vi "Interpolate 2D Scattered_Gradient.vi"(0 "X(Tri) In":dbl[][](array[numeric]), 1 "point number":i32, 5 "Y(Tri) In":dbl[][](array[numeric]), 7 "Z(Tri) In":dbl[][](array[numeric]), 9 "Area":dbl[](array[numeric]), 11 "Triangles":i32[][](array[numeric])) -> (4 "X(Tri) Out":dbl[][](array[numeric]), 6 "Y(Tri) Out":dbl[][](array[numeric]), 8 "Z(Tri) Out":dbl[][](array[numeric]), 10 "gx":dbl[][](array[numeric]), 15 "gy":dbl[][](array[numeric]))   [LabVIEW 2017, in "NI_AAL_Interpolation.lvlib"]
uses:
  <vilib>/gmath/NI_AAL_Interpolation.lvlib
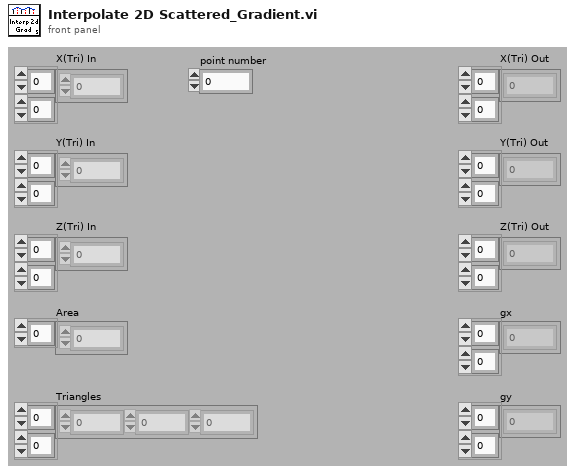
[diagram p1: front panel]
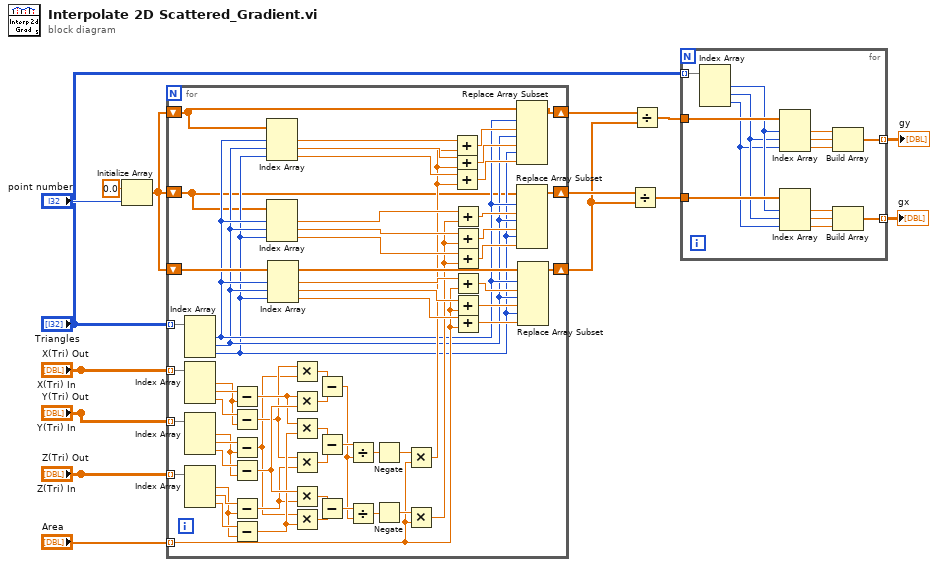
[diagram p0: block diagram]
diagram:
  n1 = Initialize Array(0.0 ("element"), "point number") -> (w12:dbl[])
  n2 = for {
    tunnel: "X(Tri) In" -> [w77] mode=indexing
    tunnel: "Y(Tri) In" -> [w76] mode=indexing
    tunnel: "Z(Tri) In" -> [w75] mode=indexing
    tunnel: "Triangles" -> [w48] mode=indexing
    tunnel: "Area" -> [w29] mode=indexing
    shift-right: [w23] -> w11
    shift-left: w12 -> [w24]
    shift-right: [w30] -> w10
    shift-left: w12 -> [w16]
    shift-right: [w41] -> w9
    shift-left: w12 -> [w42]
    n3 = Index Array(array=w48) -> (element #1=w19:i32, element #2=w18:i32, element #3=w17:i32)  [unwired: 3 in]
    n4 = Index Array(array=w77) -> (element #1=w72:dbl, element #2=w74:dbl, element #3=w73:dbl)  [unwired: 3 in]
    n5 = Index Array(array=w76) -> (element #1=w69:dbl, element #2=w71:dbl, element #3=w70:dbl)  [unwired: 3 in]
    n6 = Index Array(array=w75) -> (element #1=w66:dbl, element #2=w68:dbl, element #3=w67:dbl)  [unwired: 3 in]
    n7 = Subtract(x=w74, y=w72) -> (x-y=w54:dbl)
    n8 = Subtract(x=w73, y=w72) -> (x-y=w53:dbl)
    n9 = Subtract(x=w71, y=w69) -> (x-y=w51:dbl)
    n10 = Subtract(x=w70, y=w69) -> (x-y=w61:dbl)
    n11 = Subtract(x=w68, y=w66) -> (x-y=w52:dbl)
    n12 = Subtract(x=w67, y=w66) -> (x-y=w55:dbl)
    n13 = Index Array(array=w24, index #1=w19, index #2=w18, index #3=w17) -> (element #1=w28:dbl, element #2=w27:dbl, element #3=w26:dbl)
    n14 = Index Array(array=w16, index #1=w19, index #2=w18, index #3=w17) -> (element #1=w37:dbl, element #2=w36:dbl, element #3=w35:dbl)
    n15 = Index Array(array=w42, index #1=w19, index #2=w18, index #3=w17) -> (element #1=w45:dbl, element #2=w44:dbl, element #3=w43:dbl)
    n16 = Multiply(x=w53, y=w51) -> (x*y=w59:dbl)
    n17 = Multiply(x=w54, y=w61) -> (x*y=w60:dbl)
    n18 = Multiply(x=w54, y=w55) -> (x*y=w63:dbl)
    n19 = Multiply(x=w53, y=w52) -> (x*y=w62:dbl)
    n20 = Multiply(x=w61, y=w52) -> (x*y=w65:dbl)
    n21 = Multiply(x=w51, y=w55) -> (x*y=w64:dbl)
    n22 = Subtract(x=w59, y=w60) -> (x-y=w56:dbl)
    n23 = Subtract(x=w63, y=w62) -> (x-y=w58:dbl)
    n24 = Subtract(x=w65, y=w64) -> (x-y=w57:dbl)
    n25 = Divide(x=w58, y=w56) -> (x/y=w49:dbl)
    n26 = Divide(x=w57, y=w56) -> (x/y=w50:dbl)
    n27 = Negate(x=w49) -> (-x=w47:dbl)
    n28 = Negate(x=w50) -> (-x=w46:dbl)
    n29 = Multiply(x=w47, y=w29) -> (x*y=w25:dbl)
    n30 = Multiply(x=w46, y=w29) -> (x*y=w34:dbl)
    n31 = Add(x=w28, y=w25) -> (x+y=w22:dbl)
    n32 = Add(x=w27, y=w25) -> (x+y=w21:dbl)
    n33 = Add(x=w26, y=w25) -> (x+y=w20:dbl)
    n34 = Add(x=w37, y=w34) -> (x+y=w33:dbl)
    n35 = Add(x=w36, y=w34) -> (x+y=w32:dbl)
    n36 = Add(x=w35, y=w34) -> (x+y=w31:dbl)
    n37 = Add(x=w45, y=w29) -> (x+y=w40:dbl)
    n38 = Add(x=w44, y=w29) -> (x+y=w39:dbl)
    n39 = Add(x=w43, y=w29) -> (x+y=w38:dbl)
    n40 = Replace Array Subset(array=w24, new element #1=w22, index #1=w19, new element #2=w21, index #2=w18, new element #3=w20, index #3=w17) -> (w23:dbl[])
    n41 = Replace Array Subset(array=w16, new element #1=w33, index #1=w19, new element #2=w32, index #2=w18, new element #3=w31, index #3=w17) -> (w30:dbl[])
    n42 = Replace Array Subset(array=w42, new element #1=w40, index #1=w19, new element #2=w39, index #2=w18, new element #3=w38, index #3=w17) -> (w41:dbl[])
  }
  n43 = Divide(x=w10, y=w9) -> (x/y=w1:dbl[])
  n44 = Divide(x=w11, y=w9) -> (x/y=w8:dbl[])
  n45 = for {
    tunnel: "Triangles" -> [w89] mode=indexing
    tunnel: w1 -> [w90]
    tunnel: w8 -> [w91]
    tunnel: [w79] -> w2 mode=indexing
    tunnel: [w78] -> w3 mode=indexing
    n46 = Index Array(array=w89) -> (element #1=w88:i32, element #2=w87:i32, element #3=w86:i32)  [unwired: 3 in]
    n47 = Index Array(array=w91, index #1=w88, index #2=w87, index #3=w86) -> (element #1=w85:dbl, element #2=w84:dbl, element #3=w83:dbl)
    n48 = Index Array(array=w90, index #1=w88, index #2=w87, index #3=w86) -> (element #1=w82:dbl, element #2=w81:dbl, element #3=w80:dbl)
    n49 = Build Array(w85, w84, w83) -> (w79:dbl[])
    n50 = Build Array(w82, w81, w80) -> (w78:dbl[])
  }
  "gx" <- w3
  "gy" <- w2
  "X(Tri) Out" <- "X(Tri) In"
  "Y(Tri) Out" <- "Y(Tri) In"
  "Z(Tri) Out" <- "Z(Tri) In"
